vi "Date Server Queue_B.vi"(2 "new value":refnum<k5>, 3 "set queue? (F: de-queue)":bool) -> (0 "value":refnum<k5>, 1 "valid?":bool)   [LabVIEW 2011]
doc: "Functional Global Variable that stores each of the TCP connections made to the Data Server.vi into array of refnums.\n\n<B>Note:</B> SubVI intended for use with Data & Time Server.vi located in the TCP library."
panel:
  in  "empty":refnum<k5>
  # "Note: Intended for use with \"Multiple Connections - Server.vi\""
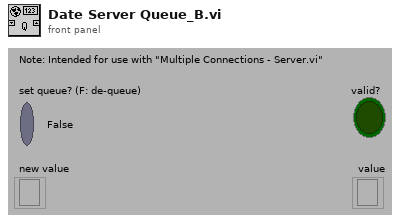
[diagram p1: front panel]
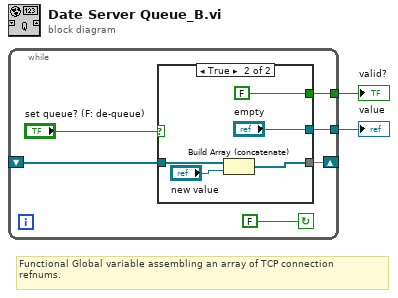
[diagram p0: block diagram]
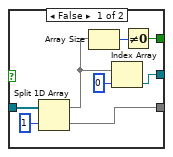
[diagram p2: hidden frame]
diagram:
  # "Functional Global variable assembling an array of TCP connection\nrefnums."
  n1 = while {
    tunnel: [w4] -> w1
    tunnel: [w5] -> w2
    shift-left: _ -> [w7]
    shift-right: [w8] -> _
    stop <- FALSE continue-if-true
    n2 = case shown="True" "set queue? (F: de-queue)" {
      tunnel: [w14 w20] -> w8
      tunnel: w7 -> [w16 w19]
      tunnel: [w11 "empty"] -> w5
      tunnel: [w9 FALSE] -> w4
      frame False {
        n3 = Split 1D Array(array=w16, index=1) -> (first subarray=w12:refnum<k5>[], second subarray=w14:refnum<k5>[])
        n4 = Array Size(array=w12) -> (size(s)=w10:i32)
        n5 = Index Array(array=w12, index=0) -> (element=w11:refnum<k5>)
        n6 = Not Equal To 0?(x=w10) -> (x != 0?=w9:bool)
      }
      frame True {
        n7 = Build Array (concatenate)(w19, "new value") -> (w20:refnum<k5>[])
      }
    }
  }
  "valid?" <- w1
  "value" <- w2
